vi "New Enumerating Connection Hanlder.vi"(8 "error in (no error)":errorcluster, 9 "connection count":refnum<data-value>, 10 "Connection Handler":refnum<class "Connection Handler.lvclass">) -> (0 "error out":errorcluster, 3 "Enumerating Connection Handler out":refnum<class "Enumerating Connection Handler.lvclass">)   [LabVIEW 2019, in "Enumerating Connection Handler.lvclass"]
uses:
  Enumerating Connection Handler.lvclass
  Connection Handler/Connection Handler.lvclass
  Enumerating Connection Handler.lvclass/Enumerating Connection Handler.ctl
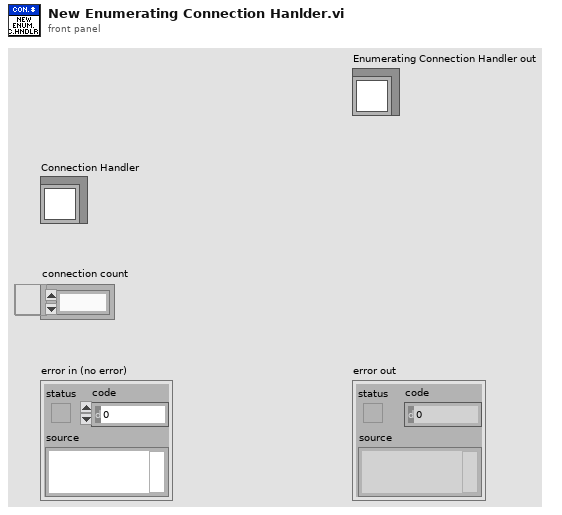
[diagram p1: front panel]
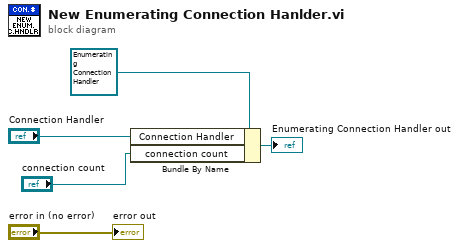
[diagram p0: block diagram]
diagram:
  n1 = Bundle By Name(cluster=refnum<class "Enumerating Connection Handler.lvclass"> refnum ("Enumerating Connection Handler in"), "Connection Handler"="Connection Handler", "connection count"="connection count") -> (→"Enumerating Connection Handler out":refnum<class "Enumerating Connection Handler.lvclass">)
  "error out" <- "error in (no error)"
